vi "main.vi"(8 "Error in":errorcluster) -> (0 "error out":errorcluster)   [LabVIEW 2018, in "Error Handler.lvlib"]
doc: "The main VI of the module."
uses:
  Error Handler.lvlib
  vi/Module Queue Actions.ctl
  ctl/Module State--enum.ctl
  Common/Common.lvlib
  Common/ctl/Stop all modules states--enum.ctl
  ctl/Error source--enum.ctl
  Common/ctl/Error to pass.ctl
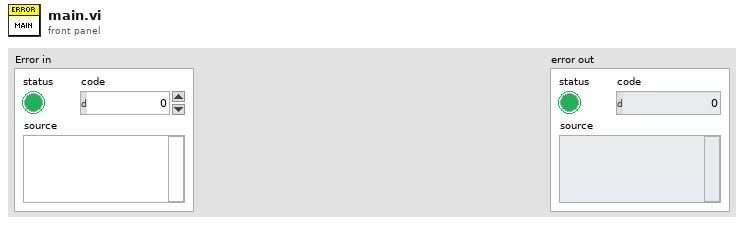
[diagram p1: front panel]
types:
  T1 = typedef "Error Handler.lvlib/Module Queue Actions.ctl" = enum16{"Create", "Get", "Destroy"}
  T2 = typedef "Common.lvlib/Stop all modules states--enum.ctl" = enum16{"Create", "Get", "Send 'Stop all' Message", "Destroy"}
  T3 = typedef "Error Handler.lvlib/Module State--enum.ctl" = enum16{"Init", "Error", "Idle", "Close", "Handle External Error", "Log to file"}
  T4 = typedef "Common.lvlib/Error source--enum.ctl" = enum16{"Display Console", "User Console", "Sensor Interface IO", "Process Step", "Other"}
  T5 = typedef "Common.lvlib/Error to pass.ctl" = cluster{"Error source":T4, "Error":errorcluster}
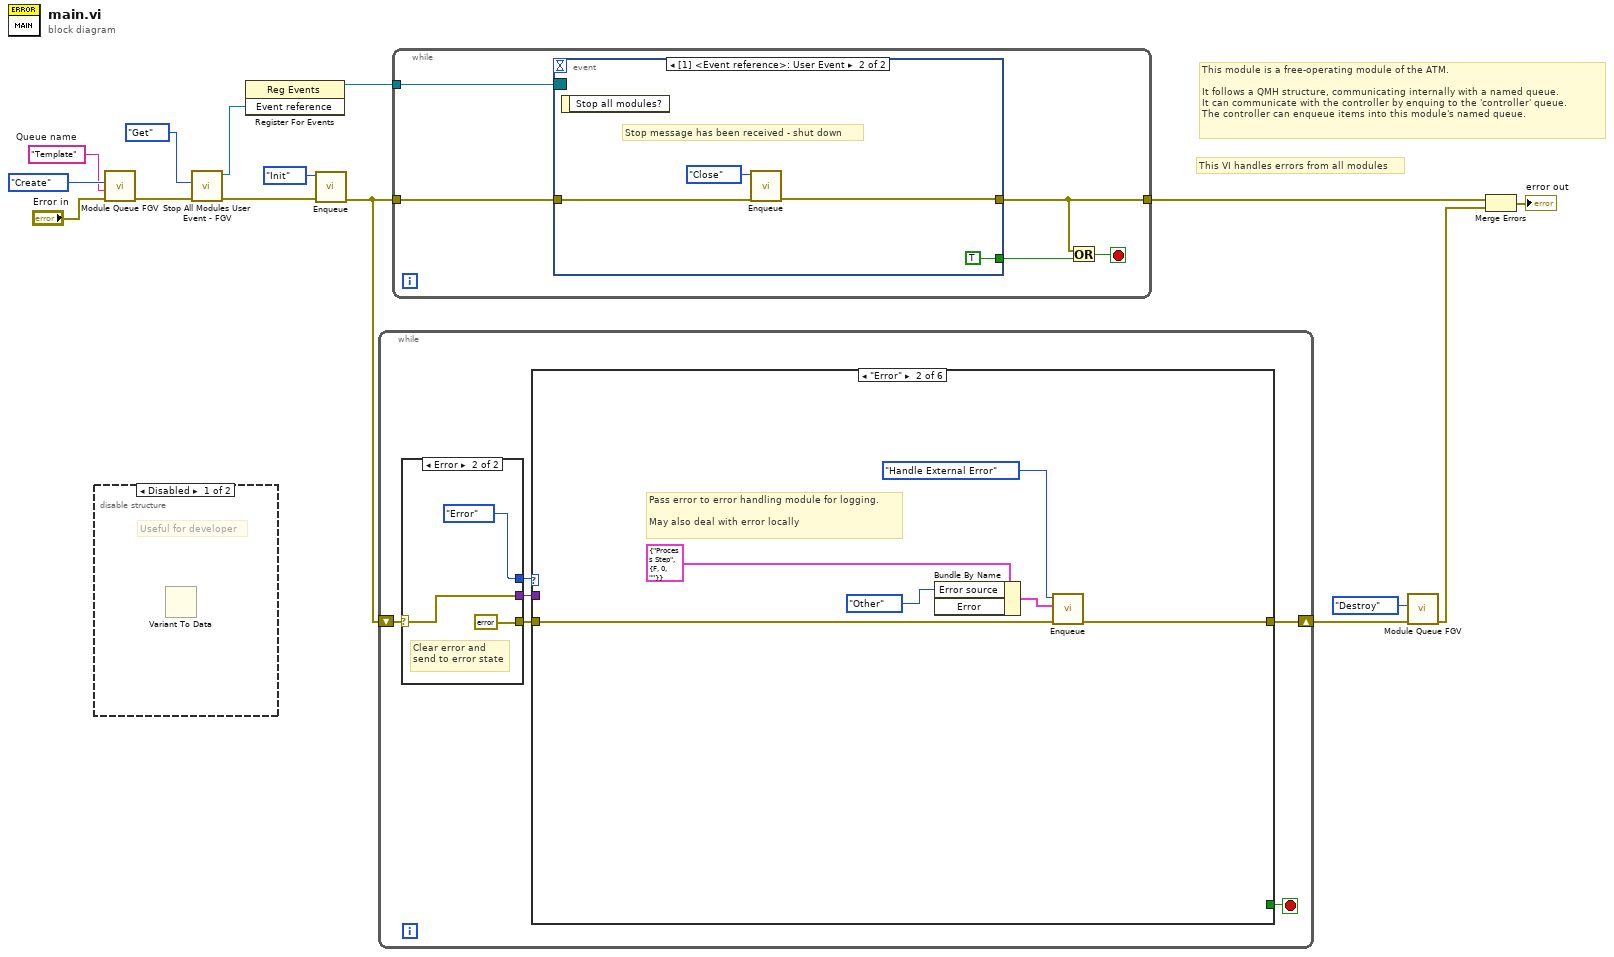
[diagram p0: block diagram]
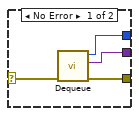
[diagram p3: hidden frame]
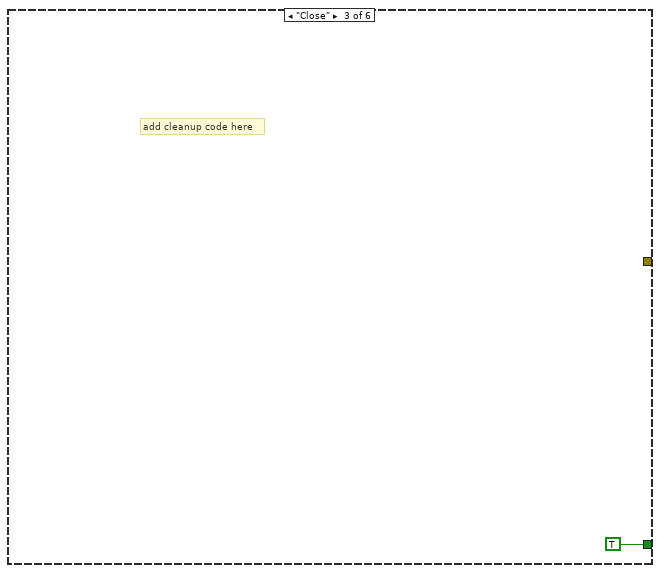
[diagram p5: hidden frame]
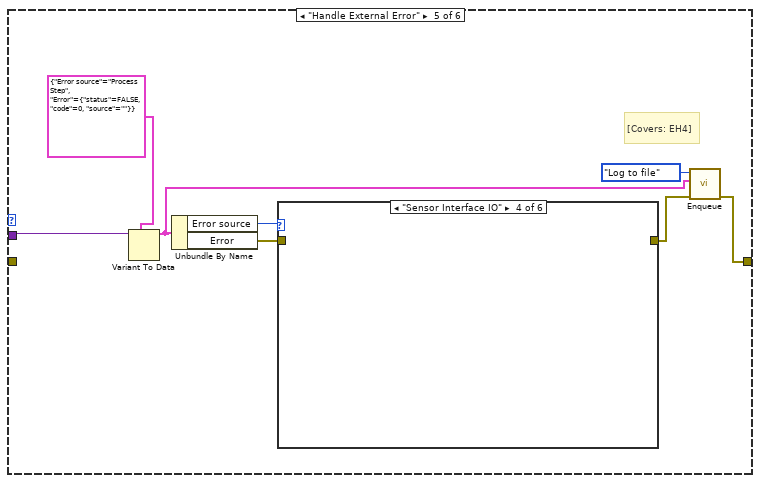
[diagram p7: hidden frame]
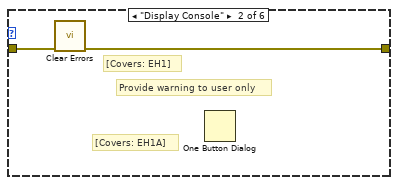
[diagram p9: hidden frame]
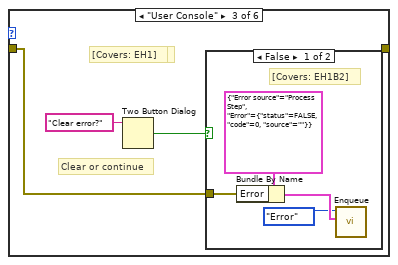
[diagram p10: hidden frame]
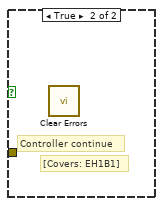
[diagram p11: hidden frame]
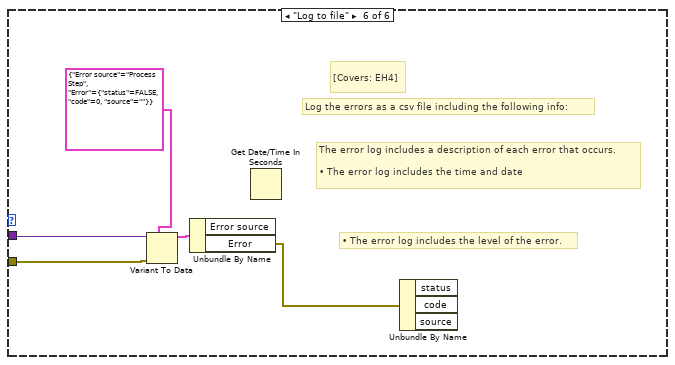
[diagram p14: hidden frame]
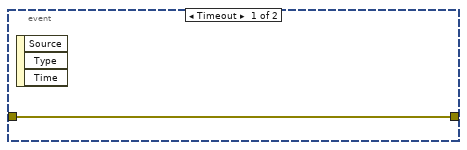
[diagram p15: hidden frame]
diagram:
  w14 = "Template"  # Queue name
  # "This VI handles errors from all modules"
  # "This module is a free-operating module of the ATM.\n\nIt follows a QMH structure, communicating internally with a named queue.\nIt can communicate with the controller by enquing to the 'controller' queue.\nThe controller can enqueue items into this module's named queue."
  n1 = disable-structure shown="Disabled" {
    frame Disabled {
      # "Useful for developer"
      n2 = Variant To Data() -> ()  [unwired: 3 in, 2 out]
    }
    frame Enabled {
    }
  }
  n3 = call "Module Queue FGV.vi"("Error in"="Error in", "Queue name"=w14, "Module Queue Actions"=Module_Queue_Actions."Create") -> ("error out"=w9:errorcluster)  [unwired: 7 in, 1 out]
  n4 = call "Stop All Modules User Event - FGV.vi"("error in"=w9, "Action"=Stop_all_modules_states--enum."Get") -> ("error out"=w8:errorcluster, "Event reference"=w11:refnum<user-event>)  [unwired: 8 in]
  n5 = register-events(w11) -> (reference out=w10:refnum<event-registration>)  [unwired: 2 in, 1 out]
  n6 = call "Enqueue.vi"("error in (no error)"=w8, "State"=Module_State--enum."Init") -> ("error out"=w7:errorcluster)  [unwired: 9 in]
  n7 = while {
    shift-right: [w16] -> w5
    shift-left: w7 -> [w18]
    stop <- w17 stop-if-true
    n8 = case shown="Error" w18 {
      selector: w18 -> [w22 w27]
      tunnel: [w25 Module_State--enum."Error" ("State")] -> w21
      tunnel: [w24 w27] -> w20
      tunnel: [w23 errorcluster {"status"=FALSE, "code"=0, "source"=""} ("error out")] -> w19
      frame No Error {
        n9 = call "Dequeue.vi"("error in (no error)"=w22) -> ("error out"=w23:errorcluster, "Data"=w24:variant, "State"=w25:T3)  [unwired: 8 in]
      }
      frame Error {
        # "Clear error and\nsend to error state"
      }
    }
    n10 = case shown="\"Error\"" w21 {
      tunnel: w20 -> [_ _ _ _ w43 w55]
      tunnel: w19 -> [_ w29 _ _ _ w54]
      tunnel: [_ _ TRUE _ _ _] -> w17
      tunnel: [_ w30 _ _ w38 _] -> w16
      frame "Init", Default {
      }
      frame "Error" {
        # "Pass error to error handling module for logging.\n\nMay also deal with error locally"
        n11 = Bundle By Name(cluster=T5 {"Error source"=enum."Process Step", "Error"={"status"=FALSE, "code"=0, "source"=""}} ("Error to pass"), "Error source"=Error_source--enum."Other") -> (w32:T5)  [unwired: 1 in]
        n12 = call "Enqueue.vi"("error in (no error)"=w29, "Data"=w32, "State"=Module_State--enum."Handle External Error") -> ("error out"=w30:errorcluster)  [unwired: 8 in]
      }
      frame "Close" {
        # "add cleanup code here"
      }
      frame "Idle" {
      }
      frame "Handle External Error" {
        # "[Covers: EH4]"
        n13 = Variant To Data(type=T5 {"Error source"=enum."Process Step", "Error"={"status"=FALSE, "code"=0, "source"=""}}, Variant=w43) -> (data=w36:T5)  [unwired: 1 in, 1 out]
        n14 = Unbundle By Name(w36) -> ("Error source"=w41:T4, "Error"=w40:errorcluster)
        n15 = case shown="\"Sensor Interface IO\"" w41 {
          tunnel: w40 -> [_ w45 w46 _ _ _]
          tunnel: [_ w44 _ _ _ _] -> w37
          frame Default {
          }
          frame "Display Console" {
            # "[Covers: EH1A]"
            # "Provide warning to user only"
            # "[Covers: EH1]"
            n16 = call <vilib>:"Clear Errors.vi"("error in (no error)"=w45) -> ("error out"=w44:errorcluster)  [unwired: 5 in, 1 out]
            n17 = One Button Dialog() -> ()  [unwired: 2 in, 1 out]
          }
          frame "User Console" {
            # "Clear or continue"
            # "[Covers: EH1B]"
            # "[Covers: EH1]"
            n18 = Two Button Dialog(message="Clear error?") -> (T button?=w48:bool)  [unwired: 2 in]
            n19 = case shown="False" w48 {
              tunnel: w46 -> [w49 _]
              frame False {
                # "[Covers: EH1B2]"
                n20 = Bundle By Name(cluster=T5 {"Error source"=enum."Process Step", "Error"={"status"=FALSE, "code"=0, "source"=""}}, "Error"=w49) -> (w51:T5)
                n21 = call "Enqueue.vi"("Data"=w51, "State"=Module_State--enum."Error") -> ()  [unwired: 9 in, 1 out]
              }
              frame True {
                # "[Covers: EH1B1]"
                # "Controller continue"
                n22 = call <vilib>:"Clear Errors.vi"() -> ()  [unwired: 6 in, 2 out]
              }
            }
          }
          frame "Sensor Interface IO" {
          }
          frame "Process Step" {
          }
          frame "Other" {
          }
        }
        n23 = call "Enqueue.vi"("error in (no error)"=w37, "Data"=w36, "State"=Module_State--enum."Log to file") -> ("error out"=w38:errorcluster)  [unwired: 8 in]
      }
      frame "Log to file" {
        # "Log the errors as a csv file including the following info:"
        # "• The error log includes the level of the error."
        # "The error log includes a description of each error that occurs.\n\n• The error log includes the time and date"
        # "[Covers: EH4]"
        n24 = Variant To Data(error in=w54, type=T5 {"Error source"=enum."Process Step", "Error"={"status"=FALSE, "code"=0, "source"=""}}, Variant=w55) -> (data=w56:T5)  [unwired: 1 out]
        n25 = Unbundle By Name(w56) -> ("Error"=w53:errorcluster)  [unwired: 1 out]
        n26 = Get Date/Time In Seconds() -> ()  [unwired: 1 out]
        n27 = Unbundle By Name(w53) -> ()  [unwired: 3 out]
      }
    }
  }
  n28 = while {
    tunnel: w7 -> [w62]
    tunnel: [w59] -> w3
    tunnel: w10 -> [w61]
    stop <- w60 stop-if-true
    n29 = event shown="[1] <Event reference>: User Event" {
      selector: w61 -> [_ _]
      dyn-events: _ -> [_ _]
      timeout: _ -> [_ _]
      tunnel: w62 -> [w63 w67]
      tunnel: [w63 w66] -> w59
      tunnel: [_ TRUE] -> w58
      event Timeout {
        n30 = event-data() -> ()  [unwired: 1 in, 3 out]
      }
      event User Event {
        # "Stop message has been received - shut down"
        n31 = event-data() -> ()  [unwired: 1 in, 1 out]
        n32 = call "Enqueue.vi"("error in (no error)"=w67, "State"=Module_State--enum."Close") -> ("error out"=w66:errorcluster)  [unwired: 9 in]
      }
    }
    n33 = Or(x=w59, y=w58) -> (x .or. y?=w60:bool)
  }
  n34 = call "Module Queue FGV.vi"("Error in"=w5, "Module Queue Actions"=Module_Queue_Actions."Destroy") -> ("error out"=w4:errorcluster)  [unwired: 8 in, 1 out]
  n35 = Merge Errors(w3, w4) -> (→"error out":errorcluster)
